vi "Disconnect.vi"(8 "error in (no error)":errorcluster, 11 "connection ID":refnum<k5>) -> (0 "error out":errorcluster)   [LabVIEW 2020, in "DAQIO MQTT.lvlib"]
doc: "Disconnects from an MQTT broker server.\n\n© 2015 - daq.io, LLC - Peter Adelhardt"
uses:
  DAQIO MQTT.lvlib
  Controls/MessageType.ctl
  Controls/Connection FGV Actions.ctl
  Controls/Connection Status FGV Actions.ctl
  Controls/Connection Return Codes.ctl
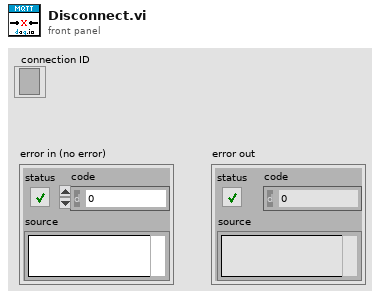
[diagram p1: front panel]
types:
  T1 = typedef "DAQIO MQTT.lvlib/Connection Return Codes.ctl" = enum16{"Connection accepted", "Connection refused: unacceptable protocol version", "Connection refused: identifier rejected", "Connection refused: Server unavailable", "Connection refused: bad user name or password", "Connection refused: not authorized"}
  T2 = typedef "DAQIO MQTT.lvlib/Connection Status FGV Actions.ctl" = enum16{"Get", "Set"}
  T3 = typedef "DAQIO MQTT.lvlib/Connection FGV Actions.ctl" = enum16{"Get", "Set", "Delete"}
  T4 = typedef "DAQIO MQTT.lvlib/MessageType.ctl" = enum32{"Reserved", "CONNECT", "CONNACK", "PUBLISH", "PUBACK", "PUBREC", "PUBREL", "PUBCOMP", "SUBSCRIBE", "SUBACK", "UNSUBSCRIBE", "UNSUBACK", "PINGREQ", "PINGRESP", "DISCONNECT", "Reserved2"}
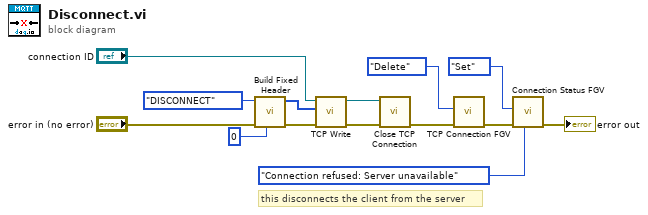
[diagram p0: block diagram]
diagram:
  # "this disconnects the client from the server"
  n1 = call "Build Fixed Header.vi"("Remaining Length"=u32 0, "error in (no error)"="error in (no error)", "MessageType"=MessageType."DISCONNECT") -> ("error out"=w11:errorcluster, "Fixed Header"=w10:u8[])  [unwired: 7 in]
  n2 = call "TCP Write.vi"("error in (no error)"=w11, "data in"=w10, "connection ID"="connection ID") -> ("error out"=w7:errorcluster, "connection ID out"=w8:refnum<k5>)  [unwired: 6 in, 1 out]
  n3 = call "Close TCP Connection.vi"("error in (no error)"=w7, "connection ID"=w8) -> ("error out"=w6:errorcluster)  [unwired: 8 in, 1 out]
  n4 = call "TCP Connection FGV.vi"("error in"=w6, "Command"=Connection_FGV_Actions."Delete") -> ("error out"=w4:errorcluster)  [unwired: 8 in, 1 out]
  n5 = call "Connection Status FGV.vi"("Connection Status in"=Connection_Return_Codes."Connection refused: Server unavailable", "error in"=w4, "Command"=Connection_Status_FGV_Actions."Set") -> ("error out"=→"error out":errorcluster)  [unwired: 7 in, 1 out]
